vi "Change Setting.vi"(8 "error in (no error)":errorcluster, 10 "Change setting mode":T1, 11 "Toggle 8 (niDig) in":refnum<class "Toggle 8 (niDig).lvclass">) -> (0 "error out":errorcluster, 1 "Changes":cluster{"Name":string, "Value":string}[](array[cluster]), 2 "Last setting":bool, 3 "Toggle 8 (niDig) out":refnum<class "Toggle 8 (niDig).lvclass">)   [LabVIEW 2020, in "Toggle 8 (niDig).lvclass"]
uses:
  Toggle 8 (niDig).lvclass
  Controls/Change setting mode enum.ctl
  niDigital.lvclass
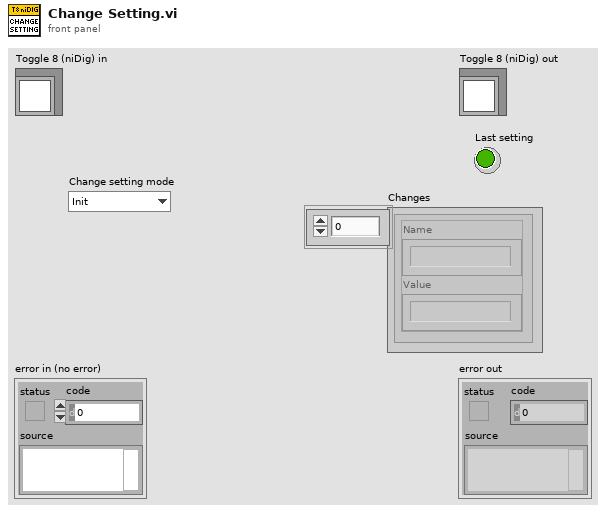
[diagram p1: front panel]
types:
  T1 = typedef "niDigital.lvclass/Change setting mode enum.ctl" = enum16{"Init", "Next", "Reset"}
  T2 = cluster{"USID":u8, "Write Address":u8, "Write Data Array":u8[]}[]
  T3 = cluster{"USID":u8, "Write Address":u8, "Write Data Array":u8[]}
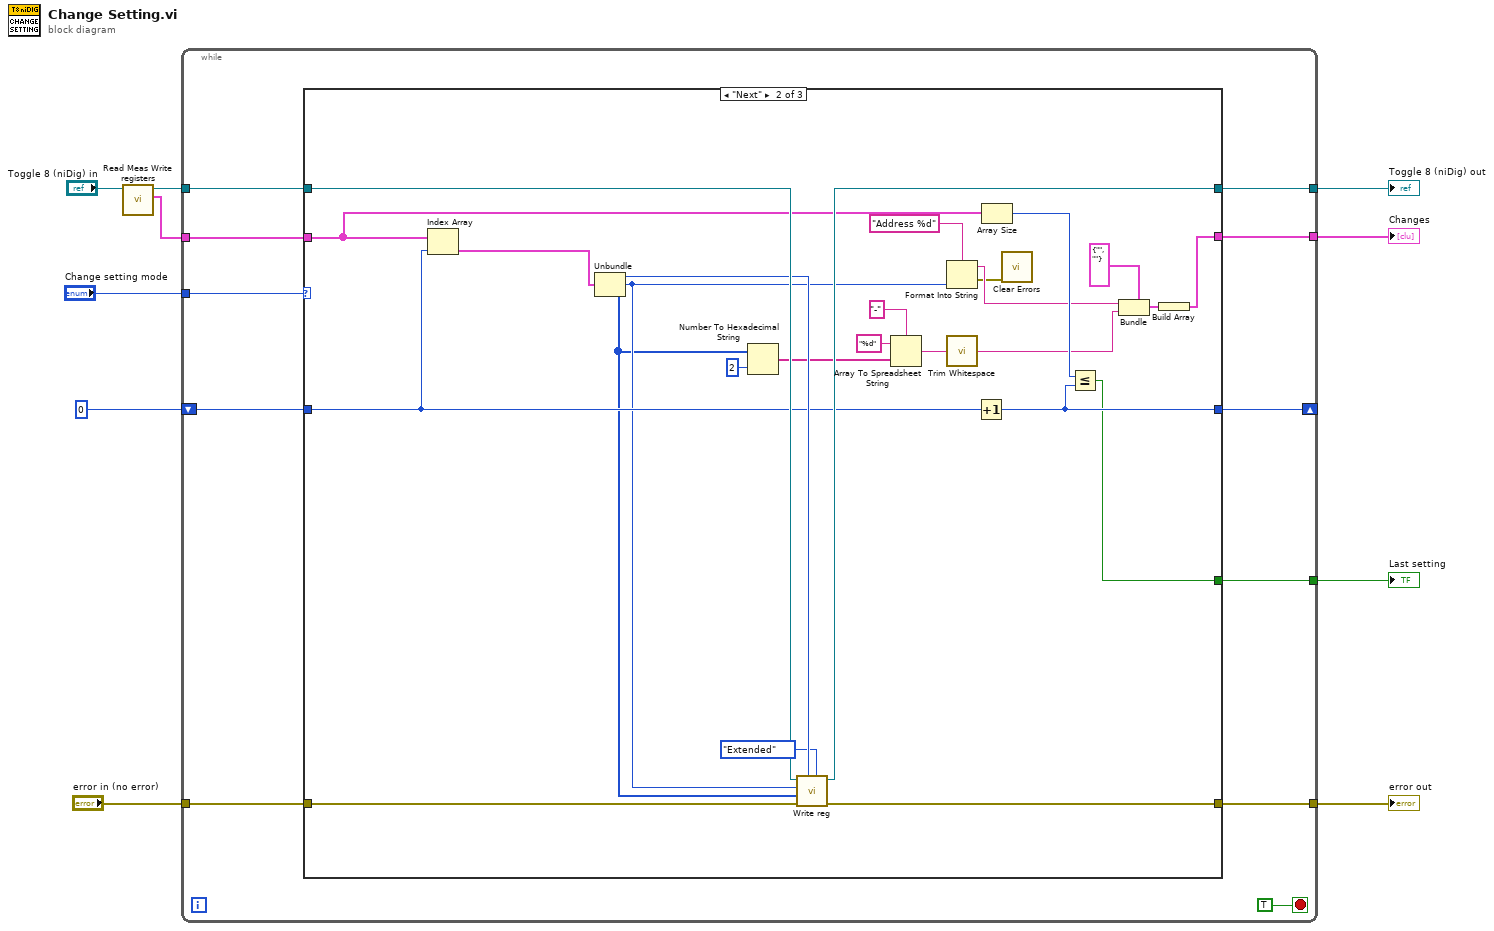
[diagram p0: block diagram]
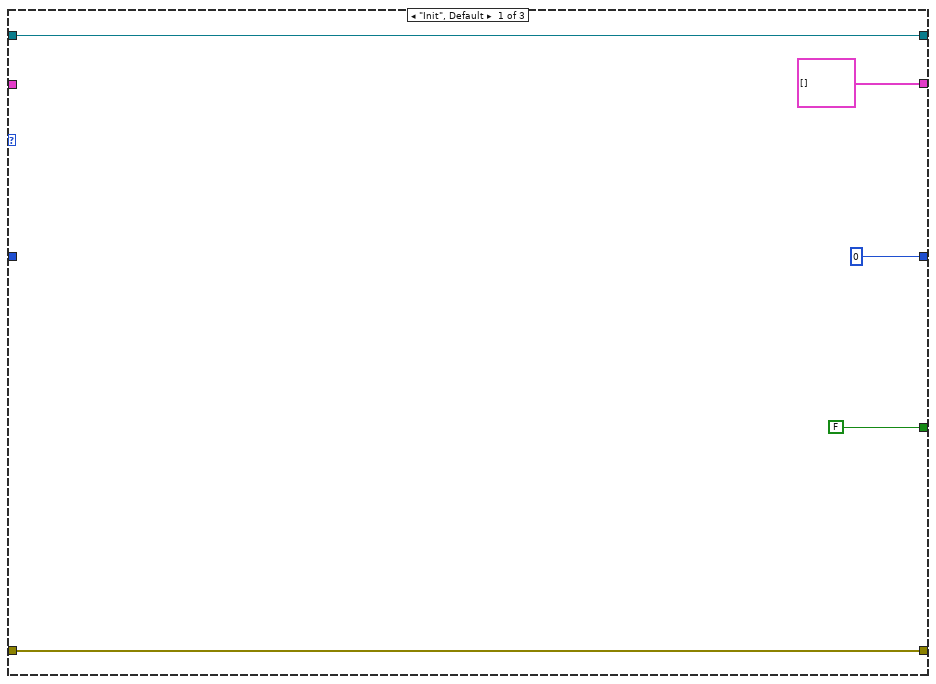
[diagram p2: hidden frame]
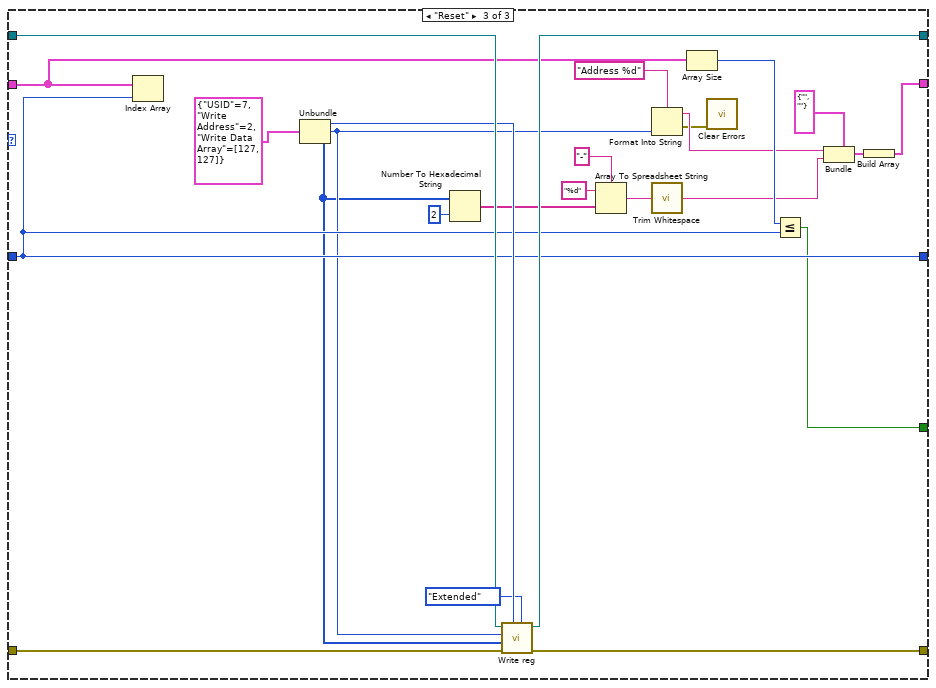
[diagram p3: hidden frame]
diagram:
  n1 = call-dynamic "Read Meas Write registers.vi"("Toggle 8 (niDig) in"="Toggle 8 (niDig) in") -> ("Meas Write registers"=w1:T2, "Toggle 8 (niDig) out"=w2:refnum<class "Toggle 8 (niDig).lvclass">)  [unwired: 9 in]
  n2 = while {
    tunnel: "Change setting mode" -> [w20]
    tunnel: "error in (no error)" -> [w19]
    tunnel: [w18] -> w9
    tunnel: [w17] -> w8
    tunnel: [w16] -> w7
    tunnel: [w15] -> w6
    shift-right: [w14] -> _
    shift-left: 0 -> [w13]
    tunnel: w2 -> [w12]
    tunnel: w1 -> [w11]
    stop <- TRUE ("stop") stop-if-true
    n3 = case shown="\"Next\"" w20 {
      tunnel: w19 -> [w24 w49 w75]
      tunnel: [w24 w48 w74] -> w18
      tunnel: [cluster{"Name":string, "Value":string}[] [] ("Changes") w39 w66] -> w17
      tunnel: [w25 w47 w73] -> w16
      tunnel: w12 -> [w25 w51 w77]
      tunnel: [FALSE w42 w69] -> w15
      tunnel: [0 w44 w72] -> w14
      tunnel: w13 -> [_ w46 w72]
      tunnel: w11 -> [_ w45 w71]
      frame "Init", Default {
      }
      frame "Next" {
        n4 = Index Array(array=w45, index=w46) -> (element=w52:T3)
        n5 = Unbundle(w52) -> ("USID"=w50:u8, "Write Address"=w33:u8, "Write Data Array"=w28:u8[])
        n6 = Number To Hexadecimal String(1:i16 2 ("width (-)"), 2:w28) -> (0:w27:string[])
        n7 = call-dynamic "Write reg.vi"("Write type"=enum16{"Normal", "Extended", "Extended Cycle"}."Extended", "Write USID"=w50, "error in (no error)"=w49, "Write Data"=w28, "Write Address"=w33, "niDigital in"=w51) -> ("error out"=w48:errorcluster, "niDigital out"=w47:refnum<class "Toggle 8 (niDig).lvclass">)  [unwired: 4 in]
        n8 = Array To Spreadsheet String(delimiter (Tab)="-", array=w27, 3:"%d" ("format string")) -> (spreadsheet string=w36:string)
        n9 = Format Into String(format string="Address %d", w33) -> (resulting string=w32:string, error out=w31:errorcluster)  [unwired: 2 in]
        n10 = call <vilib>:"Trim Whitespace.vi"("string"=w36) -> ("trimmed string"=w35:string)  [unwired: 1 in]
        n11 = Increment(x=w46) -> (x+1=w44:i32)
        n12 = Array Size(array=w45) -> (size(s)=w43:i32)
        n13 = call <vilib>:"Clear Errors.vi"("error in (no error)"=w31) -> ()  [unwired: 5 in, 2 out]
        n14 = Less Or Equal?(x=w43, y=w44) -> (x <= y?=w42:bool)
        n15 = Bundle(cluster=cluster{"Name":string, "Value":string} {"Name"="", "Value"=""} ("Change"), "Name"=w32, "Value"=w35) -> (w40:cluster{"Name":string, "Value":string})
        n16 = Build Array(w40) -> (w39:cluster{"Name":string, "Value":string}[])
      }
      frame "Reset" {
        n17 = Index Array(array=w71, index=w72) -> ()  [unwired: 1 out]
        n18 = Unbundle(T3 {"USID"=7, "Write Address"=2, "Write Data Array"=[127, 127]} ("cluster")) -> ("USID"=w76:u8, "Write Address"=w60:u8, "Write Data Array"=w55:u8[])
        n19 = Number To Hexadecimal String(1:i16 2 ("width (-)"), 2:w55) -> (0:w54:string[])
        n20 = call-dynamic "Write reg.vi"("Write type"=enum16{"Normal", "Extended", "Extended Cycle"}."Extended", "Write USID"=w76, "error in (no error)"=w75, "Write Data"=w55, "Write Address"=w60, "niDigital in"=w77) -> ("error out"=w74:errorcluster, "niDigital out"=w73:refnum<class "Toggle 8 (niDig).lvclass">)  [unwired: 4 in]
        n21 = Array To Spreadsheet String(delimiter (Tab)="-", array=w54, 3:"%d" ("format string")) -> (spreadsheet string=w63:string)
        n22 = Format Into String(format string="Address %d", w60) -> (resulting string=w59:string, error out=w58:errorcluster)  [unwired: 2 in]
        n23 = call <vilib>:"Trim Whitespace.vi"("string"=w63) -> ("trimmed string"=w62:string)  [unwired: 1 in]
        n24 = Array Size(array=w71) -> (size(s)=w70:i32)
        n25 = call <vilib>:"Clear Errors.vi"("error in (no error)"=w58) -> ()  [unwired: 5 in, 2 out]
        n26 = Less Or Equal?(x=w70, y=w72) -> (x <= y?=w69:bool)
        n27 = Bundle(cluster=cluster{"Name":string, "Value":string} {"Name"="", "Value"=""} ("Change"), "Name"=w59, "Value"=w62) -> (w67:cluster{"Name":string, "Value":string})
        n28 = Build Array(w67) -> (w66:cluster{"Name":string, "Value":string}[])
      }
    }
  }
  "error out" <- w9
  "Toggle 8 (niDig) out" <- w7
  "Changes" <- w8
  "Last setting" <- w6
